vi "Set Field Value and Rate.vi"(0 "IP Address":string="128.174.165.97", 1 "Target Field X mT":dbl, 2 "Target Field Y mT":dbl, 3 "Target Field Z mT":dbl, 11 "error in (no error)":errorcluster, 12 "Ramp Rate mT per s":dbl=0.1) -> (15 "error out":errorcluster)   [LabVIEW 2024]
panel:
  out "Current Z FIeld mT":dbl=0.059
  out "Current Y Field mT":dbl
  out "Current X Field mT":dbl
  out "Response String":string
  # "Before use, turn on the magnet supply and switch heater,\nOpen the VRM software"
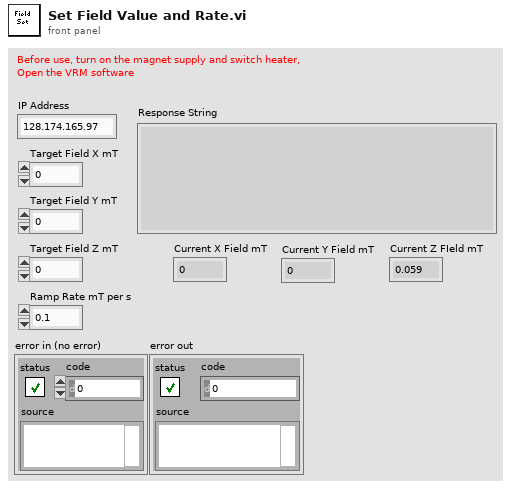
[diagram p1: front panel]
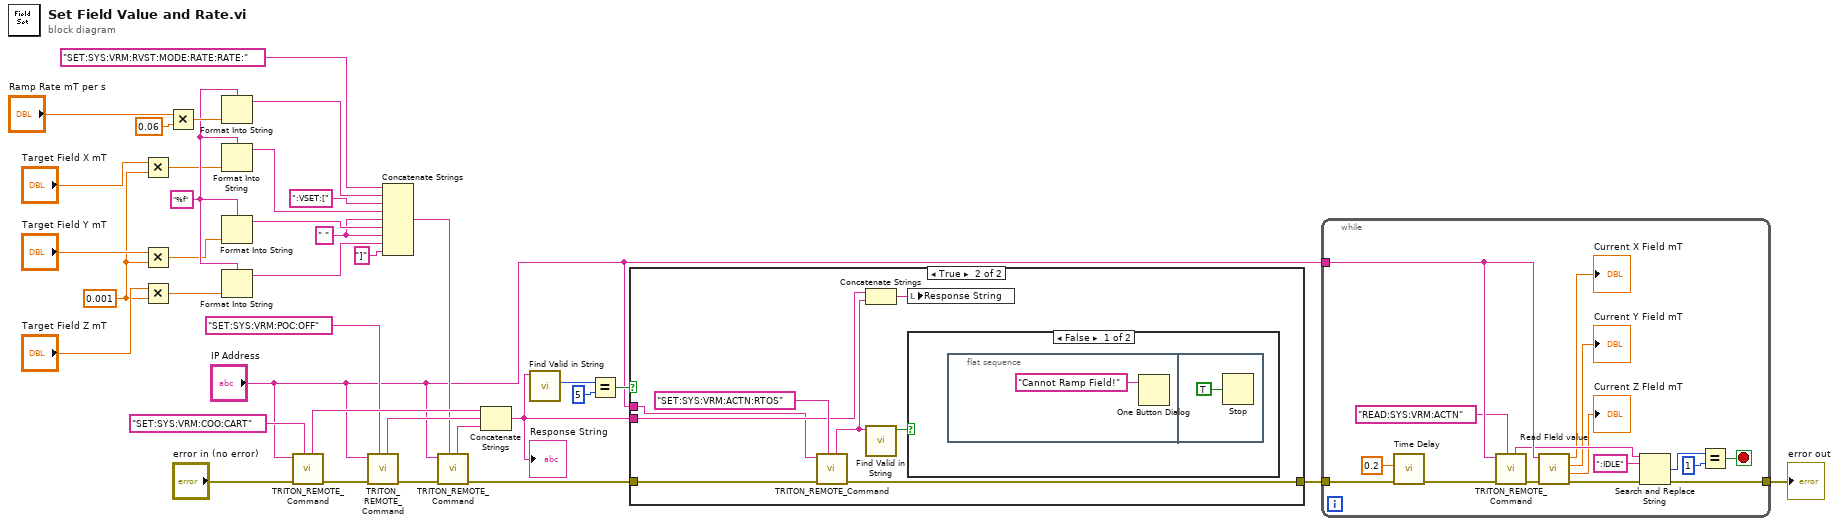
[diagram p0: block diagram]
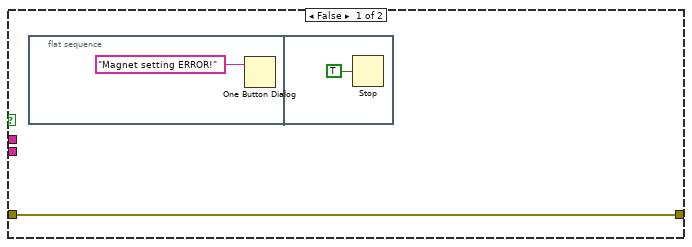
[diagram p2: hidden frame]
diagram:
  w11 = 0.001 ("y")
  w15 = " " ("string")
  w21 = "%f" ("format string")
  n1 = Multiply(x="Target Field X mT", y=w11) -> (x*y=w14:dbl)
  n2 = Multiply(x="Target Field Y mT", y=w11) -> (x*y=w13:dbl)
  n3 = Multiply(x="Target Field Z mT", y=w11) -> (x*y=w12:dbl)
  n4 = Multiply(x="Ramp Rate mT per s", y=0.06) -> (x*y=w26:dbl)
  n5 = Format Into String(format string=w21, w26) -> (resulting string=w24:string)  [unwired: 2 in, 1 out]
  n6 = Format Into String(format string=w21, w14) -> (resulting string=w18:string)  [unwired: 2 in, 1 out]
  n7 = Format Into String(format string=w21, w13) -> (resulting string=w17:string)  [unwired: 2 in, 1 out]
  n8 = Format Into String(format string=w21, w12) -> (resulting string=w16:string)  [unwired: 2 in, 1 out]
  n9 = call "TRITON_REMOTE_Command.vi"("Command to send"="SET:SYS:VRM:COO:CART", "error in (no error)"="error in (no error)", "IP Address"="IP Address") -> ("error out"=w33:errorcluster, "Response String"=w34:string)  [unwired: 6 in, 1 out]
  n10 = call "TRITON_REMOTE_Command.vi"("Command to send"="SET:SYS:VRM:POC:OFF", "error in (no error)"=w33, "IP Address"="IP Address") -> ("error out"=w30:errorcluster, "Response String"=w31:string)  [unwired: 6 in, 1 out]
  n11 = Concatenate Strings("SET:SYS:VRM:RVST:MODE:RATE:RATE:" ("Command to send"), w24, ":VSET:[" ("string"), w18, w15, w17, w15, w16, "]" ("string")) -> (w10:string)
  n12 = call "TRITON_REMOTE_Command.vi"("Command to send"=w10, "error in (no error)"=w30, "IP Address"="IP Address") -> ("error out"=w5:errorcluster, "Response String"=w29:string)  [unwired: 6 in, 1 out]
  n13 = Concatenate Strings(w34, w31, w29) -> (w4:string)
  "Response String" <- w4
  n14 = call "Find Valid in String.vi"("string"=w4) -> ("number of findings"=w8:i32)  [unwired: 9 in, 1 out]
  n15 = Equal?(x=w8, y=5) -> (x = y?=w6:bool)
  n16 = case shown="True" w6 {
    tunnel: "IP Address" -> [_ w40]
    tunnel: w5 -> [w37 w47]
    tunnel: w4 -> [_ w45]
    tunnel: [w37 w41] -> w2
    frame False {
      n17 = flat-sequence {
        frame #0 {
          n18 = One Button Dialog(message="Magnet setting ERROR!") -> ()  [unwired: 1 in, 1 out]
        }
        frame #1 {
          n19 = Stop(stop? (T)=TRUE) -> ()
        }
      }
    }
    frame True {
      n20 = call "TRITON_REMOTE_Command.vi"("Command to send"="SET:SYS:VRM:ACTN:RTOS", "error in (no error)"=w47, "IP Address"=w40) -> ("error out"=w41:errorcluster, "Response String"=w43:string)  [unwired: 6 in, 1 out]
      n21 = Concatenate Strings(w45, w43) -> (w44:string)
      n22 = call "Find Valid in String.vi"("string"=w43) -> ("Found"=w42:bool)  [unwired: 9 in, 1 out]
      n23 = local write "Response String"(w44) -> ()
      n24 = case shown="False" w42 {
        frame False {
          n25 = flat-sequence {
            frame #0 {
              n26 = One Button Dialog(message="Cannot Ramp Field!") -> ()  [unwired: 1 in, 1 out]
            }
            frame #1 {
              n27 = Stop(stop? (T)=TRUE) -> ()
            }
          }
        }
        frame True {
        }
      }
    }
  }
  n28 = while {
    tunnel: "IP Address" -> [w65]
    tunnel: w2 -> [w52]
    tunnel: [w53] -> w1
    stop <- w57 stop-if-true
    n29 = call "Time Delay"("error in (no error)"=w52, "Delay Time (s)"=0.2) -> ("error out"=w51:errorcluster)  [unwired: 9 in]
    n30 = call "TRITON_REMOTE_Command.vi"("Command to send"="READ:SYS:VRM:ACTN", "error in (no error)"=w51, "IP Address"=w65) -> ("error out"=w63:errorcluster, "Response String"=w62:string)  [unwired: 6 in, 1 out]
    n31 = call "Read FIeld value.vi"("error in (no error)"=w63, "IP Address"=w65) -> ("error out"=w60:errorcluster, "Z FIeld mT"=→"Current Z FIeld mT":dbl, "Y Field mT"=→"Current Y Field mT":dbl, "X Field mT"=→"Current X Field mT":dbl)  [unwired: 6 in]
    n32 = Search and Replace String(input string=w62, search string=":IDLE", error in=w60) -> (number of replacements=w59:i32, error out=w53:errorcluster)  [unwired: 5 in, 2 out]
    n33 = Equal?(x=w59, y=1) -> (x = y?=w57:bool)
  }
  "error out" <- w1
